vi "CH4_Rx.vi"() -> ()   [LabVIEW 2018]
uses:
  Stream/Stream.lvclass
  RxTx/RxTx.lvclass
  Stream/Stream.lvclass/Stream.ctl
panel:
  in  "RxTx.lvclass":refnum<class "RxTx.lvclass">
  in  "Stream.lvclass":refnum<class "Stream.lvclass">
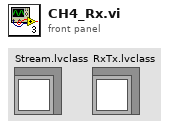
[diagram p1: front panel]
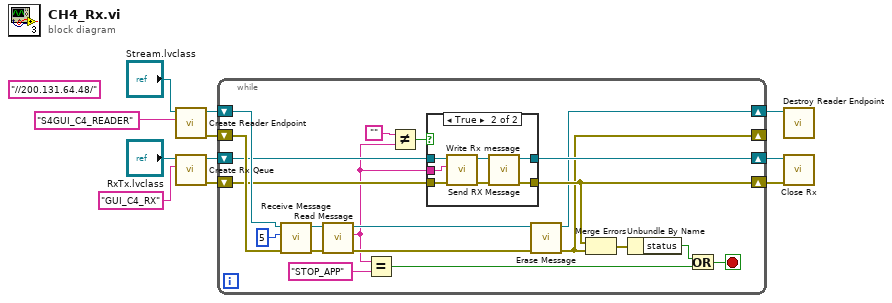
[diagram p0: block diagram]
diagram:
  (unwired) "//200.131.64.48/" ("Reader Name")
  n1 = call "Create Reader Endpoint.vi"("reader name"="S4GUI_C4_READER", "Stream in"="Stream.lvclass") -> ("error out"=w9:errorcluster, "Stream out"=w10:refnum<class "Stream.lvclass">)  [unwired: 8 in]
  n2 = call "Create Rx Qeue.vi"("Reader Name"="GUI_C4_RX", "RxTx in"="RxTx.lvclass") -> ("error out"=w4:errorcluster, "RxTx out"=w5:refnum<class "RxTx.lvclass">)  [unwired: 8 in]
  n3 = while {
    shift-right: [w17] -> _
    shift-left: w9 -> [w31]
    shift-right: [w20] -> w8
    shift-left: w10 -> [w32]
    shift-right: [w24] -> w2
    shift-left: w4 -> [w28]
    shift-right: [w26] -> w3
    shift-left: w5 -> [w27]
    stop <- w14 stop-if-true
    n4 = call "Receive Message.vi"("error in (no error)"=w31, "timeout ms"=5, "Stream in"=w32) -> ("error out"=w29:errorcluster, "Stream out"=w30:refnum<class "Stream.lvclass">)  [unwired: 7 in]
    n5 = call "Read Message.vi"("error in (no error)"=w29, "Stream in"=w30) -> ("error out"=w19:errorcluster, "Message"=w16:string, "Stream out"=w18:refnum<class "Stream.lvclass">)  [unwired: 7 in]
    n6 = Equal?(x=w16, y="STOP_APP" ("reader name")) -> (x = y?=w12:bool)
    n7 = Not Equal?(x="", y=w16) -> (x != y?=w21:bool)
    n8 = case shown="True" w21 {
      tunnel: w28 -> [w33 w39]
      tunnel: w27 -> [w34 w38]
      tunnel: w16 -> [_ w37]
      tunnel: [w34 w36] -> w26
      tunnel: [w33 w35] -> w24
      frame False {
      }
      frame True {
        n9 = call "Write Rx message.vi"("error in (no error)"=w39, "Rx message"=w37, "RxTx in"=w38) -> ("error out"=w40:errorcluster, "RxTx out"=w41:refnum<class "RxTx.lvclass">)  [unwired: 7 in]
        n10 = call "Send RX Message.vi"("error in (no error)"=w40, "RxTx in"=w41) -> ("error out"=w35:errorcluster, "RxTx out"=w36:refnum<class "RxTx.lvclass">)  [unwired: 8 in]
      }
    }
    n11 = call "Erase Message.vi"("error in (no error)"=w19, "Stream in"=w18) -> ("error out"=w17:errorcluster, "Stream out"=w20:refnum<class "Stream.lvclass">)  [unwired: 8 in]
    n12 = Merge Errors(w24, w17) -> (w25:errorcluster)
    n13 = Unbundle By Name(w25) -> ("status"=w13:bool)
    n14 = Or(x=w13, y=w12) -> (x .or. y?=w14:bool)
  }
  n15 = call "Destroy Reader Endpoint.vi"("Stream in"=w8) -> ()  [unwired: 9 in, 2 out]
  n16 = call "Close Rx.vi"("error in (no error)"=w2, "RxTx in"=w3) -> ()  [unwired: 8 in, 2 out]
